vi "Record Nested.vi"(8 "error in (no error)":errorcluster, 10 "Nested Queue":refnum<class "Priority Message Queue.lvclass">, 11 "Actor API in":refnum<class "Actor API.lvclass">) -> (0 "error out":errorcluster, 3 "Actor API out":refnum<class "Actor API.lvclass">)   [LabVIEW 2020, in "Artifex.lvlib" / "Actor API.lvclass"]
uses:
  Actor API.lvclass
  Priority Message Queue/Priority Message Queue.lvclass
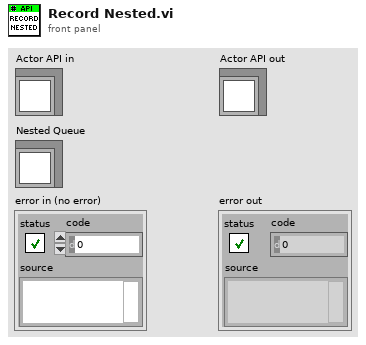
[diagram p1: front panel]
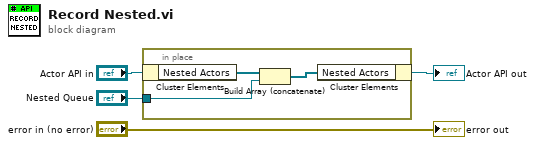
[diagram p0: block diagram]
diagram:
  n1 = in-place {
    in-place-border: "Nested Queue" -> [w6]
    n2 = in-place-cluster #1("Actor API in") -> ("Nested Actors"=w7:refnum<class "Priority Message Queue.lvclass">[])
    n3 = Build Array (concatenate)(w7, w6) -> (w5:refnum<class "Priority Message Queue.lvclass">[])
    n4 = in-place-cluster #1("Nested Actors"=w5) -> (→"Actor API out":refnum<class "Actor API.lvclass">)
  }
  "error out" <- "error in (no error)"
